vi "delete_I_think_Initialize Configuration File.vi"(8 "error in (no error)":errorcluster, 11 "Instrument.Lockin in":refnum<class "Instrument.Lockin.lvclass">) -> (0 "error out":errorcluster, 3 "Instrument.Lockin out":refnum<class "Instrument.Lockin.lvclass">)   [LabVIEW 2019, in "Instrument.Lockin.lvclass"]
uses:
  Instrument.Lockin.lvclass
  C:/Program Files (x86)/National Instruments/LabVIEW 2019/user.lib/LevyLab/Instrument Framework/SMOs/Instrument/Instrument.lvclass
  <userlib>/LevyLab/Instrument Framework/SMOs/Instrument/Instrument.lvclass
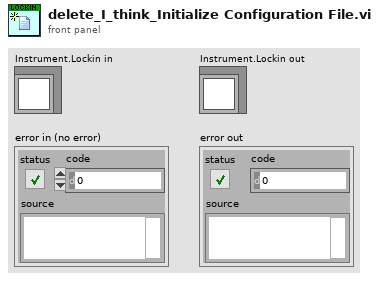
[diagram p1: front panel]
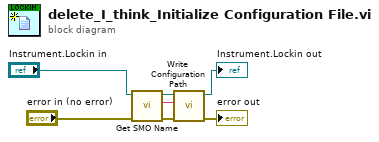
[diagram p0: block diagram]
diagram:
  n1 = call-dynamic "Get SMO Name.vi"("error in (no error)"="error in (no error)", "Instrument.Lockin"="Instrument.Lockin in") -> ("error out"=w7:errorcluster, "SMO Name"=w2:string, "Instrument.Lockin out"=w1:refnum<class "Instrument.Lockin.lvclass">)  [unwired: 7 in]
  n2 = call <userlib>:"Write Configuration Path.vi"("error in (no error)"=w7, "name or relative path"=w2, "Instrument in"=w1) -> ("error out"=→"error out":errorcluster, "Instrument out"=→"Instrument.Lockin out":refnum<class "Instrument.Lockin.lvclass">)  [unwired: 7 in]
